vi "Read Codes.vi"(8 "error in (no error)":errorcluster, 11 "System Log in":refnum<class "System Log.lvclass">) -> (0 "error out":errorcluster, 2 "Codes":i32[](array[numeric]), 3 "System Log out":refnum<class "System Log.lvclass">)   [LabVIEW 2016, in "System Log.lvclass"]
uses:
  System Log.lvclass
  System Log.lvclass/System Log.ctl
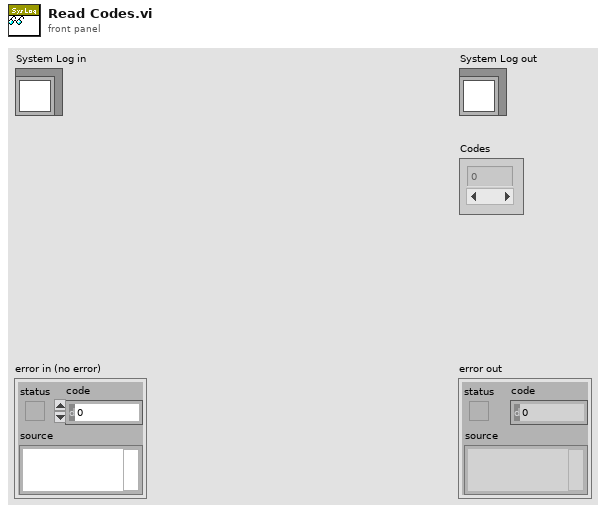
[diagram p1: front panel]
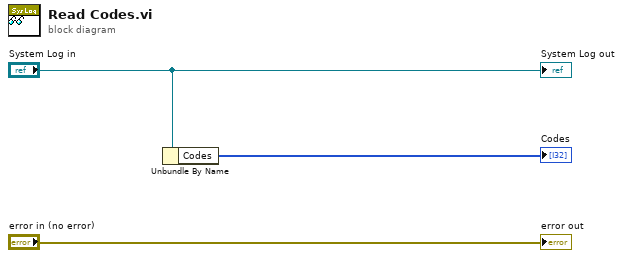
[diagram p0: block diagram]
diagram:
  n1 = Unbundle By Name("System Log in") -> ("Codes"=→"Codes":i32[])
  "error out" <- "error in (no error)"
  "System Log out" <- "System Log in"
